vi "Driver Install.vi"(7 "app reference":refnum<vi>, 8 "error in (no error)":errorcluster, 10 "Driver Library Path":path, 11 "DriverID DriverType (\"\")":string) -> (0 "error out":errorcluster, 2 "dup Driver Library Path":path)   [LabVIEW 2011]
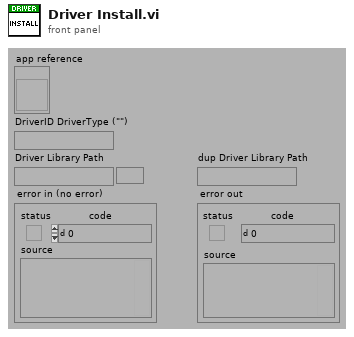
[diagram p1: front panel]
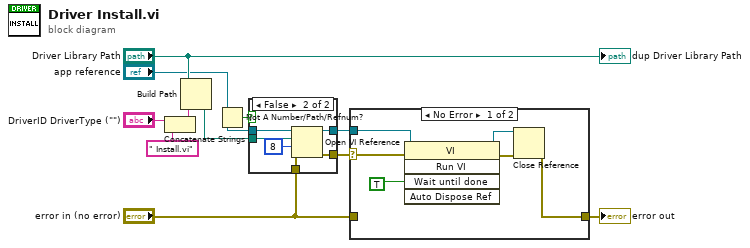
[diagram p0: block diagram]
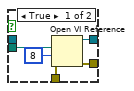
[diagram p2: hidden frame]
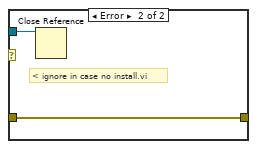
[diagram p3: hidden frame]
diagram:
  n1 = Concatenate Strings("DriverID DriverType (\"\")", " Install.vi" ("name or relative path")) -> (w4:string)
  n2 = Build Path(base path="Driver Library Path", name or relative path=w4) -> (appended path=w11:path)
  n3 = Not A Number/Path/Refnum?(number/path/refnum="app reference") -> (NaN/Path/Refnum?=w2:bool)
  n4 = case shown="False" w2 {
    tunnel: w11 -> [w16 w22]
    tunnel: [w15 w21] -> w10
    tunnel: [w13 w19] -> w8
    tunnel: "error in (no error)" -> [w12 w18]
    tunnel: "app reference" -> [_ w17]
    frame True {
      n5 = Open VI Reference(vi path=w16, options=8, error in (no error)=w12) -> (vi reference=w15:refnum<vi>, error out=w13:errorcluster)  [unwired: 3 out]
    }
    frame False {
      n6 = Open VI Reference(application reference (local)=w17, vi path=w22, options=8, error in (no error)=w18) -> (vi reference=w21:refnum<vi>, error out=w19:errorcluster)  [unwired: 2 out]
    }
  }
  n7 = case shown="No Error" w8 {
    selector: w8 -> [w23 _]
    tunnel: w10 -> [w28 w29]
    tunnel: [w25 w30] -> w9
    tunnel: "error in (no error)" -> [_ w30]
    frame No Error {
      n8 = invoke class="VI" method="Run VI"(reference=w28, error in=w23, "Wait until done"=TRUE) -> (reference out=w26:refnum<vi>, error out=w27:errorcluster)  [unwired: 2 in, 3 out]
      n9 = Close Reference(reference=w26, error in (no error)=w27) -> (error out=w25:errorcluster)
    }
    frame Error {
      # "< ignore in case no install.vi"
      n10 = Close Reference(reference=w29) -> ()  [unwired: 1 in, 1 out]
    }
  }
  "error out" <- w9
  "dup Driver Library Path" <- "Driver Library Path"
